vi "EVENT STRUCTURE.vi"() -> ()   [LabVIEW 2019]
panel:
  in  "stop":bool
  out "count":u32
  in  "increment":bool
  # "EVENT STRUCTURE"
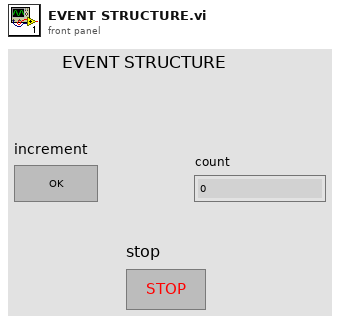
[diagram p1: front panel]
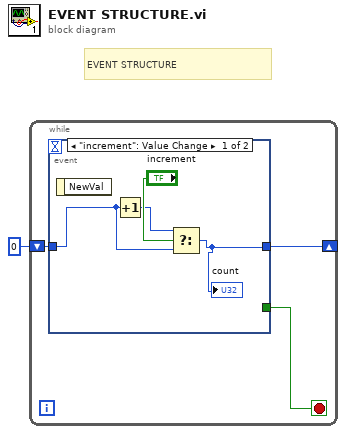
[diagram p0: block diagram]
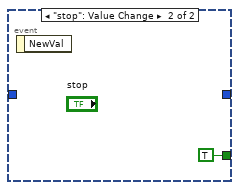
[diagram p2: hidden frame]
diagram:
  # "EVENT STRUCTURE"
  n1 = while {
    shift-right: [w4] -> _
    shift-left: u32 0 -> [w3]
    stop <- w2 stop-if-true
    n2 = event shown="[0] \"increment\": Value Change" {
      selector: _ -> [_ _]
      dyn-events: _ -> [_ _]
      timeout: _ -> [_ _]
      tunnel: [w5 _] -> w4
      tunnel: w3 -> [w6 _]
      tunnel: [_ TRUE ("stop")] -> w2
      event "increment": Value Change {
        n3 = event-data() -> ()  [unwired: 1 in, 1 out]
        n4 = Increment(x=w6) -> (x+1=w7:u32)
        n5 = Select(t=w7, s="increment", f=w6) -> (s? t:f=w5:u32)
        "count" <- w5
      }
      event "stop": Value Change {
        n6 = event-data() -> ()  [unwired: 1 in, 1 out]
      }
    }
  }
